vi "Handle WELCOME.vi"(9 "WAMP Message":T1 {"Message Codes" items=["HELLO"=1, "WELCOME"=2, "ABORT"=3, "GOODBYE"=6, "ERROR"=8, "PUBLISH"=16, "PUBLISHED"=17, "SUBSCRIBE"=32, "SUBSCRIBED"=33, "UNSUBSCRIBE"=34, "UNSUBSCRIBED"=35, "EVENT"=36, "CALL"=48, "RESULT"=59, "REGISTER"=64, "REGISTERED"=65, "UNREGISTER"=66, "UNREGISTERED"=67, "INVOCATION"=68, "YIELD"=70]}, 10 "error in (no error)":errorcluster, 11 "WAMP Client in":refnum<class "WAMP Client.lvclass">) -> (1 "Session ID":u32, 2 "error out":errorcluster, 3 "WAMP Client out":refnum<class "WAMP Client.lvclass">)   [LabVIEW 2020, in "WAMP Client.lvclass"]
uses:
  <userlib>/wamplv/WAMP Client/WAMP Client.lvclass
  <userlib>/wamplv/WAMP Client/TypeDef/WAMP Received Message.ctl
  <userlib>/wamplv/WAMP Message Codes.ctl
  81aa3083-7749-3644-b591-d0aa62dd8321.vi
  <vilib>/JDP Science/JSONtext/JSON text to Variant.vi
  <vilib>/JDP Science/JSONtext/LVClass Serializer/JSONtext LVClass Serializer.lvclass
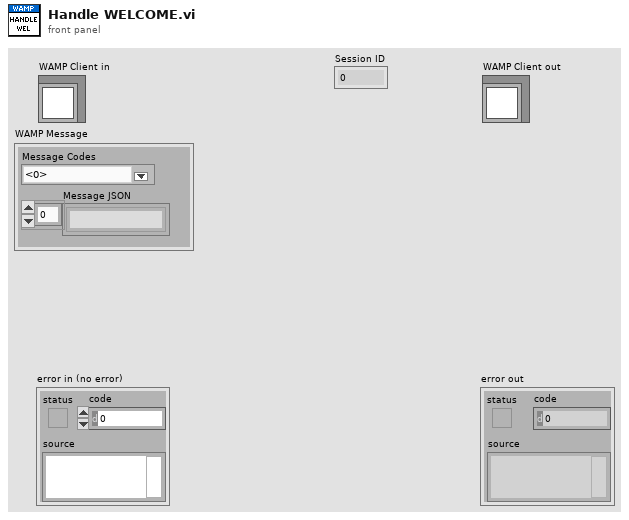
[diagram p1: front panel]
types:
  T1 = typedef "WAMP Client.lvclass/WAMP Received Message.ctl" = cluster{"Message JSON":string[], "Message Codes":T2}
  T2 = typedef "WAMP Client.lvclass/WAMP Message Codes.ctl" = u16
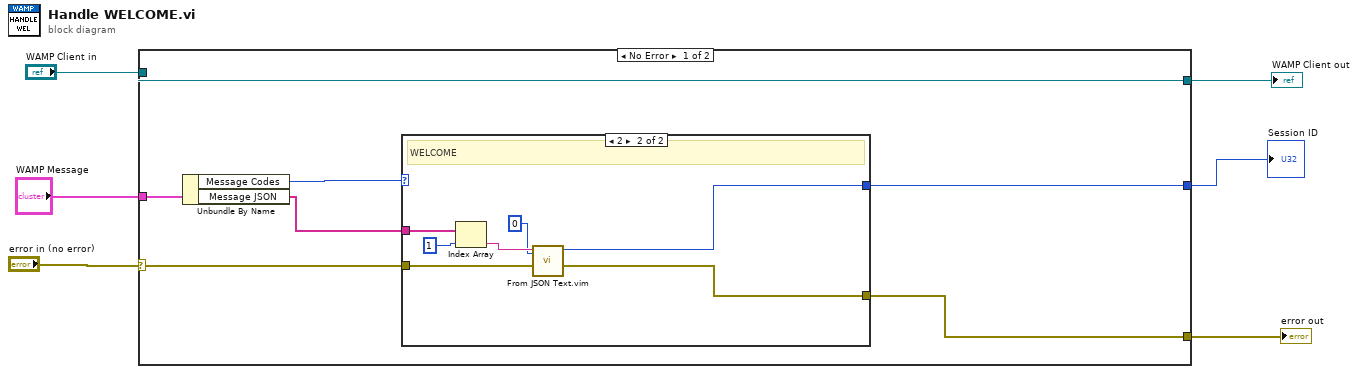
[diagram p0: block diagram]
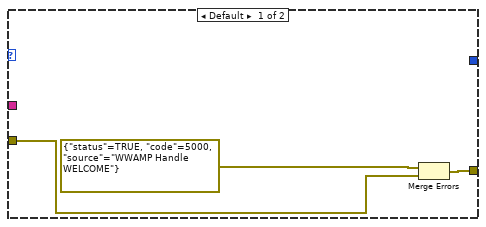
[diagram p2: hidden frame]
diagram:
  n1 = case shown="No Error" "error in (no error)" {
    selector: "error in (no error)" -> [w8 w25]
    tunnel: [w12 w25] -> w5
    tunnel: [w13 w24] -> w3
    tunnel: "WAMP Client in" -> [w13 w24]
    tunnel: [w11 _] -> w2
    tunnel: "WAMP Message" -> [w10 _]
    frame No Error {
      n2 = Unbundle By Name(w10) -> ("Message Codes"=w9:T2, "Message JSON"=w7:string[])
      n3 = case shown="2" w9 {
        tunnel: [w15 w20] -> w12
        tunnel: [_ w19] -> w11
        tunnel: w8 -> [w14 w18]
        tunnel: w7 -> [_ w17]
        frame Default {
          n4 = Merge Errors(errorcluster {"status"=TRUE, "code"=5000, "source"="WWAMP Handle WELCOME"} ("error in"), w14) -> (w15:errorcluster)
        }
        frame 2 {
          # "WELCOME"
          n5 = Index Array(array=w17, index=1) -> (element=w22:string)
          n6 = call "From JSON Text.vim"("Data Type and Default Value"=u32 0, "error in (no error)"=w18, "JSON"=w22) -> ("error out"=w20:errorcluster, "Data out"=w19:u32)  [unwired: 7 in]
        }
      }
    }
    frame Error {
    }
  }
  "error out" <- w5
  "WAMP Client out" <- w3
  "Session ID" <- w2
